vi "ex_4b.vi"() -> ()   [LabVIEW 2020]
panel:
  out "Array":i32[][](array[numeric])
  in  "M":i32
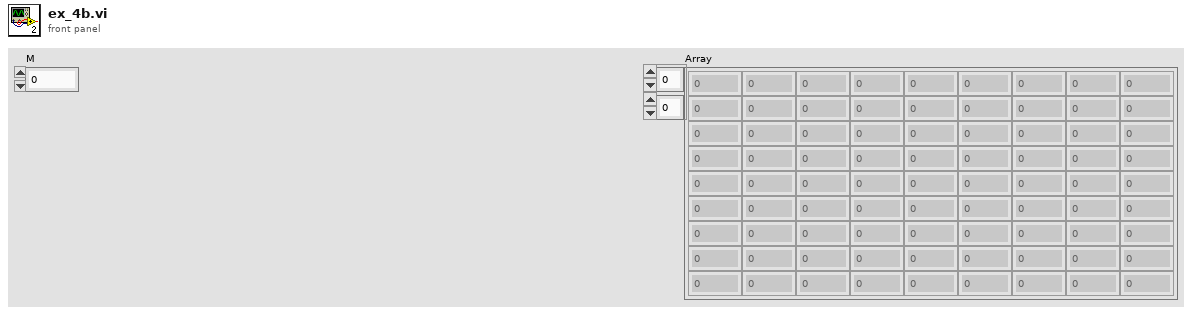
[diagram p1: front panel]
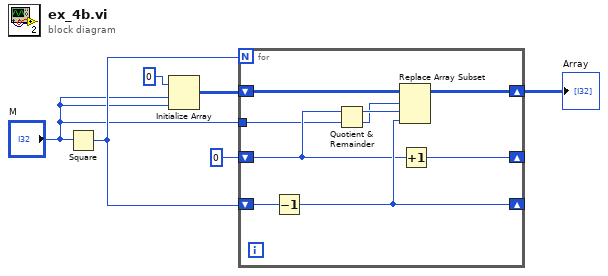
[diagram p0: block diagram]
diagram:
  n1 = Square(x="M") -> (x^2=w6:i32)
  n2 = Initialize Array(0, "M", "M") -> (w3:i32[][])
  n3 = for {
    N: w6 -> [_]
    shift-right: [w13] -> w4
    shift-left: w3 -> [w15]
    shift-right: [w9] -> _
    shift-left: w6 -> [w14]
    shift-right: [w12] -> _
    shift-left: 0 -> [w8]
    tunnel: "M" -> [w7]
    n4 = Decrement(x=w14) -> (x-1=w9:i32)
    n5 = Quotient & Remainder(x=w8, y=w7) -> (x-y*floor(x/y)=w11:i32, floor(x/y)=w10:i32)
    n6 = Replace Array Subset(array=w15, new element=w9, index (row)=w10, index (col)=w11) -> (w13:i32[][])
    n7 = Increment(x=w8) -> (x+1=w12:i32)
  }
  "Array" <- w4
